vi "WLC Fitting For OneDirectionOnly_Slope_YCC.vi"() -> ()   [LabVIEW 2014]
uses:
  SubVI/WLC-Fitting Cluster.ctl
  <vilib>/gmath/NI_Gmath.lvlib
  <vilib>/gmath/NumericalOptimization/Nonlinear Curve Fit LM formula string.vi
  <vilib>/Utility/file.llb/Write To Spreadsheet File (DBL).vi
  <vilib>/Utility/file.llb/Read From Spreadsheet File (DBL).vi
panel:
  in  "F+U data?":bool
  in  "Ready to Fit":bool
  out "Save to Path":path
  out "best nonlinear fit force":dbl[](array[numeric])
  in  "SaveName":enum16{"ForecExtension Only", "WLC Fitting"}(ring)
  in  "Save Data?":bool
  in  "Finish Fitting":bool
  out "best fit parameters":dbl[](array[numeric])
  in  "initial parameters 2":dbl[](array[numeric])=[40.0, 1150.0]
  in  "Enum":T1(ring)
  in  "initial parameters for fit K":dbl[](array[numeric])=[40.0, 1150.0]
  out "Force":dbl[](array[numeric])
  out "xDNA":dbl[](array[numeric])
  out "Fitting Cluster for indicator":T2={"cr (um)"=0.0, "yr (V)"=0.0, "trap height(nm)"=0.0, "bead radius(nm)"=520.0, "Length offset"=0.0, "Upper Force(pN)"=0.0, "cr shift (nm)"=0.0, "yr shift (mV)"=0.0, "LaserPower (mW)"=0.0, "conversion factor (V/um)"=0.0, "Stiffness (pN/nm)"=0.0154, "xDNA cut outside"=3000.0, "Lower Force(pN)"=5.0}
  in  "OneDirectionOnly?":bool=TRUE
  in  "Fitting Cluster for contorl":T3={"cr (um)"=0.0, "yr (V)"=0.0, "trap height(nm)"=300.0, "bead radius(nm)"=515.0, "Length offset"=0.0, "conversion factor (V/um)"=0.0, "Force constant (pN/nm)"=0.0154, "Force offset"=5.0, "cr shift (nm)"=0.0, "yr shift (mV)"=0.0, "LaserPower (mW)"=30.0, "Cf. Calib. Array"=[0.10341, -0.29934], "Stiffness Calib. array"=[0.0034, -0.00514]}
  in  "Tab Control":T4(tab)
  out "Stage-QPD Graph":T5(graph)
  out "Extension-Force Graph":cluster{"xDNA":dbl[], "Force":dbl[]}(graph)
  out "Extension-Force and WLC Graph":cluster{"xDNA":dbl[], "Force":dbl[]}[](graph)
  out "Cut Stage Position (um)":dbl[](array[numeric])
  out "Cut QPD (V)":dbl[](array[numeric])
  in  "Delete Outside Signal?":bool
  out "QPD signal (V)":dbl[](array[numeric])
  out "Stage Positions (um)":dbl[](array[numeric])
  in  "Load Stage-QPD data":path
  in  "QPD":dbl[](array[numeric])
  in  "Stage":dbl[](array[numeric])
  in  "T=Read data mode?\nF=Real time fit":bool=TRUE
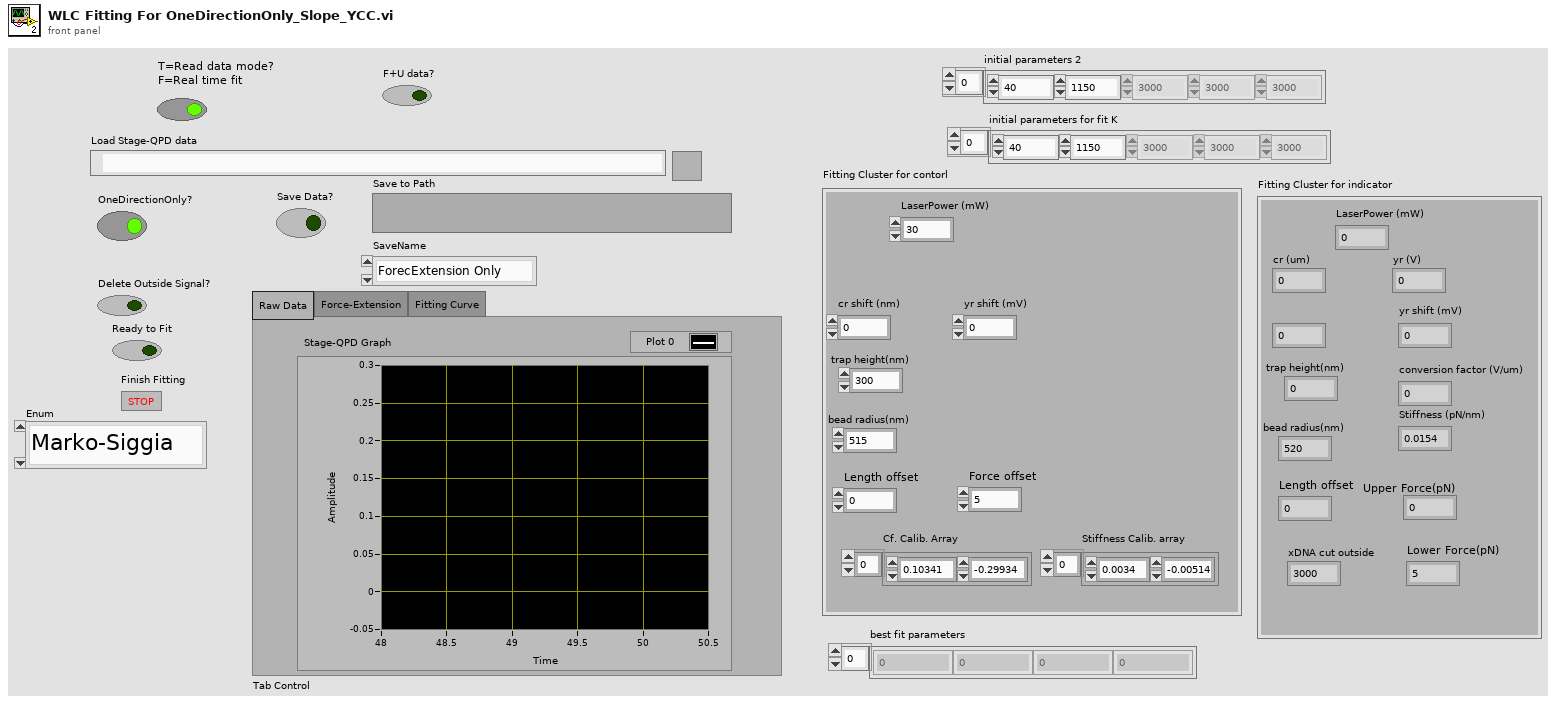
[diagram p1: front panel]
types:
  T1 = enum16{"Marko-Siggia", "modified Marko", "eWLC", "eWLC-modified M-S", "K fit eWLC-modified M-S"}
  T2 = typedef "WLC-Fitting Cluster.ctl" = cluster{"cr (um)":dbl, "yr (V)":dbl, "trap height(nm)":dbl, "bead radius(nm)":dbl, "Length offset":dbl, "Upper Force(pN)":dbl, "cr shift (nm)":dbl, "yr shift (mV)":dbl, "LaserPower (mW)":dbl, "conversion factor (V/um)":dbl, "Stiffness (pN/nm)":dbl, "xDNA cut outside":dbl, "Lower Force(pN)":dbl}
  T3 = typedef "WLC-Fitting Cluster.ctl" = cluster{"cr (um)":dbl, "yr (V)":dbl, "trap height(nm)":dbl, "bead radius(nm)":dbl, "Length offset":dbl, "conversion factor (V/um)":dbl, "Force constant (pN/nm)":dbl, "Force offset":dbl, "cr shift (nm)":dbl, "yr shift (mV)":dbl, "LaserPower (mW)":dbl, "Cf. Calib. Array":dbl[], "Stiffness Calib. array":dbl[]}
  T4 = enum32{"Raw Data", "Force-Extension", "Fitting Curve"}
  T5 = cluster{"Sorted Stage Position (um)":dbl[], "Sorted QPD (V)":dbl[]}[]
  T6 = cluster{"model":string, "Parameters":string[], "x":string}
  T7 = cluster{"Stage Positions (um)":dbl[], "QPD signal (V)":dbl[]}
  T8 = cluster{"Position Array Out":dbl[], "QPD signal Out":dbl[]}
  T9 = cluster{"Stage Positions (um)":dbl[], "QPD signal (V)":dbl[]}[]
  T10 = cluster{"Unfolded-xDNA":dbl[], "Unfolded-Force":dbl[]}
  T11 = cluster{"xDNA":dbl[], "best nonlinear fit":dbl[]}
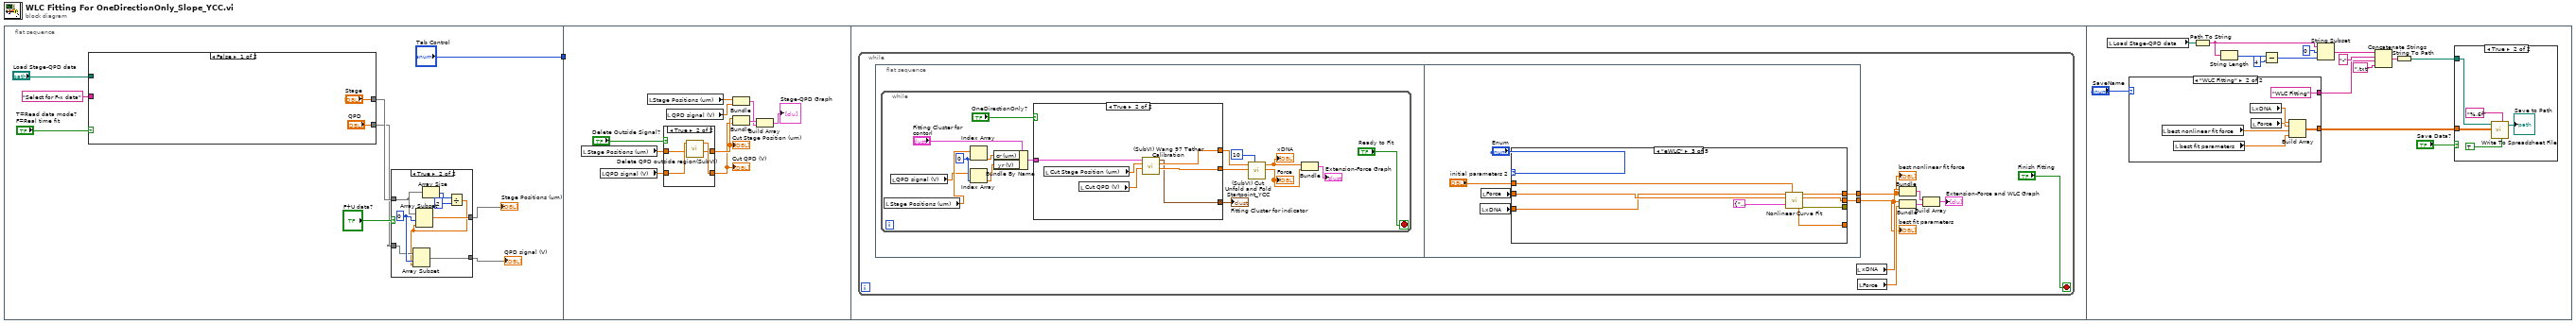
[diagram p0: block diagram]
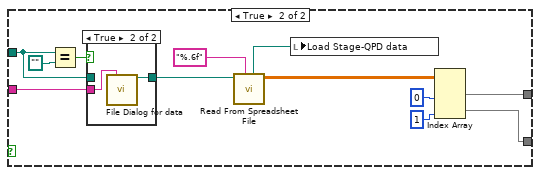
[diagram p3: hidden frame]
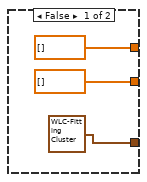
[diagram p6: hidden frame]
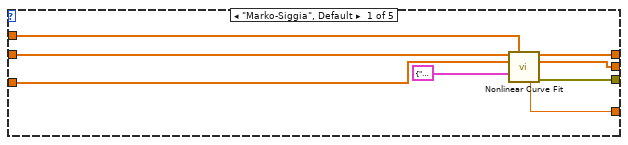
[diagram p7: hidden frame]
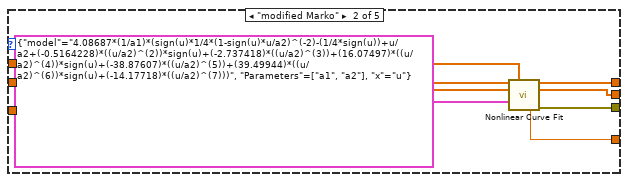
[diagram p8: hidden frame]
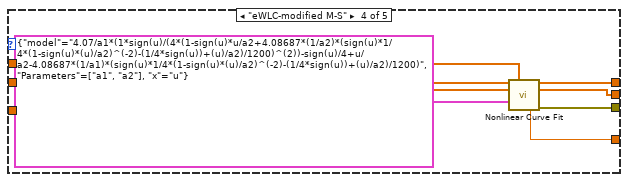
[diagram p9: hidden frame]
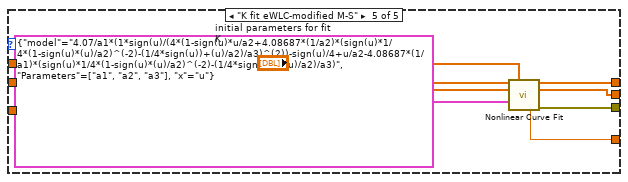
[diagram p10: hidden frame]
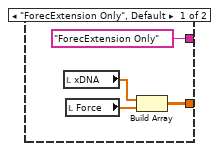
[diagram p11: hidden frame]
diagram:
  n1 = flat-sequence {
    tunnel: ["Tab Control"] -> w1
    tunnel: w1 -> [_]
    frame #0 {
      n2 = case shown="False" "T=Read data mode?\nF=Real time fit" {
        tunnel: ["QPD" w30] -> w4
        tunnel: ["Stage" w31] -> w5
        tunnel: "Select for F-x data" ("default name") -> [_ w27]
        tunnel: "Load Stage-QPD data" -> [_ w24]
        frame False {
        }
        frame True {
          n3 = Equal?(x=w24, y=path "") -> (x = y?=w25:bool)
          n4 = case shown="True" w25 {
            tunnel: [w35 w36] -> w28
            tunnel: w27 -> [_ w37]
            tunnel: w24 -> [w35 _]
            frame False {
            }
            frame True {
              n5 = call "File Dialog for data"("prompt"=w37) -> ("selected path"=w36:path)  [unwired: 11 in, 3 out]
            }
          }
          n6 = call-poly <vilib>:"Read From Spreadsheet File.vi"("format (%.3f)"="%.6f", "file path (dialog if empty)"=w28) -> ("all rows"=w34:dbl[][], "new file path (Not A Path if cancelled)"=w23:path)  [unwired: 5 in, 3 out]
          n7 = local write "Load Stage-QPD data"(w23) -> ()
          n8 = Index Array(array=w34, index (col) #1=0 ("disabled index (col)"), index (col) #2=1 ("index (col)")) -> (element #1=w31:dbl[], element #2=w30:dbl[])  [unwired: 2 in]
        }
      }
      n9 = case shown="True" "F+U data?" {
        tunnel: w5 -> [w12 w20]
        tunnel: w4 -> [w11 w15]
        tunnel: [w12 w17] -> w3
        tunnel: [w11 w13] -> w2
        frame False {
        }
        frame True {
          w16 = 0 ("index")
          n10 = Array Size(array=w20) -> (size(s)=w19:i32)
          n11 = Divide(x=w19, y=2) -> (x/y=w14:dbl)
          n12 = Array Subset(array=w15, index=w16, length=w14) -> (w13:dbl[])
          n13 = Array Subset(array=w20, index=w16, length=w14) -> (w17:dbl[])
        }
      }
      "Stage Positions (um)" <- w3
      "QPD signal (V)" <- w2
    }
    frame #1 {
      n14 = local read "Stage Positions (um)"() -> (w46:dbl[])
      n15 = local read "QPD signal (V)"() -> (w45:dbl[])
      n16 = local read "Stage Positions (um)"() -> (w44:dbl[])
      n17 = case shown="True" "Delete Outside Signal?" {
        tunnel: w45 -> [w49 w53]
        tunnel: w46 -> [w48 w52]
        tunnel: [w49 w51] -> w38
        tunnel: [w48 w50] -> w39
        frame False {
        }
        frame True {
          n18 = call "Delete QPD outside region(SubVI).vi"("Position Array In"=w52, "QPD signal In"=w53) -> ("Position Array Out"=w50:dbl[], "QPD signal Out"=w51:dbl[])  [unwired: 8 in]
        }
      }
      "Cut QPD (V)" <- w38
      "Cut Stage Position (um)" <- w39
      n19 = local read "QPD signal (V)"() -> (w43:dbl[])
      n20 = Bundle("Stage Positions (um)"=w44, "QPD signal (V)"=w43) -> (w41:T7)  [unwired: 1 in]
      n21 = Bundle("Position Array Out"=w39, "QPD signal Out"=w38) -> (w42:T8)  [unwired: 1 in]
      n22 = Build Array(w42, w41) -> (→"Stage-QPD Graph":T9)
    }
    frame #2 {
      n23 = while {
        stop <- "Finish Fitting" stop-if-true
        n24 = flat-sequence {
          tunnel: [w88] -> w55
          tunnel: [w87] -> w54
          frame #0 {
            n25 = while {
              stop <- "Ready to Fit" stop-if-true
              w75 = 0 ("index")
              n26 = local read "Stage Positions (um)"() -> (w64:dbl[])
              n27 = local read "QPD signal (V)"() -> (w63:dbl[])
              n28 = Index Array(array=w64, index=w75) -> (element=w72:dbl)
              n29 = Index Array(array=w63, index=w75) -> (element=w62:dbl)
              n30 = Bundle By Name(cluster="Fitting Cluster for contorl", "cr (um)"=w72, "yr (V)"=w62) -> (w74:T3)
              n31 = case shown="True" "OneDirectionOnly?" {
                tunnel: w74 -> [_ w86]
                tunnel: [T2 {"cr (um)"=0.0, "yr (V)"=0.0, "trap height(nm)"=0.0, "bead radius(nm)"=520.0, "Length offset"=0.0, "Upper Force(pN)"=0.0, "cr shift (nm)"=0.0, "yr shift (mV)"=0.0, "LaserPower (mW)"=0.0, "conversion factor (V/um)"=0.0, "Stiffness (pN/nm)"=0.0154, "xDNA cut outside"=3000.0, "Lower Force(pN)"=5.0} ("Fitting Cluster for contorl") w81] -> w73
                tunnel: [dbl[] [] ("xDNA") w83] -> w68
                tunnel: [dbl[] [] ("Force") w82] -> w67
                frame False {
                }
                frame True {
                  n32 = local read "Cut Stage Position (um)"() -> (w85:dbl[])
                  n33 = local read "Cut QPD (V)"() -> (w84:dbl[])
                  n34 = call "(SubVI) Wang 97 Tether Calibration.vi"("QPD signal"=w84, "Stage Position"=w85, "Fitting Cluster"=w86) -> ("Force"=w82:dbl[], "xDNA"=w83:dbl[], "output cluster"=w81:T2)  [unwired: 2 in]
                }
              }
              "Fitting Cluster for indicator" <- w73
              n35 = call "(SubVI) Cut Unfold and Fold Startpoint_YCC.vi"("number to cut"=10, "Unfolded-Force"=w67, "Unfolded-xDNA"=w68) -> ("Unfolded-Force"=w65:dbl[], "Unfolded-xDNA"=w66:dbl[])  [unwired: 5 in, 2 out]
              "xDNA" <- w66
              "Force" <- w65
              n36 = Bundle("Unfolded-xDNA"=w66, "Unfolded-Force"=w65) -> (→"Extension-Force Graph":T10)  [unwired: 1 in]
            }
          }
          frame #1 {
            n37 = local read "xDNA"() -> (w90:dbl[])
            n38 = local read "Force"() -> (w91:dbl[])
            n39 = case shown="\"eWLC\"" "Enum" {
              tunnel: "initial parameters 2" -> [w94 w107 w113 w123 _]
              tunnel: w91 -> [w99 w105 w115 w121 w131]
              tunnel: w90 -> [w93 w106 w114 w122 w130]
              tunnel: [w98 w102 w111 w117 w125] -> w88
              tunnel: [w97 w103 w112 w118 w126] -> w87
              tunnel: [w96 w104 w110 w119 w127] -> _
              tunnel: [w95 w101 w109 w120 w128] -> _
              frame "Marko-Siggia", Default {
                n40 = call-poly <vilib>:"Nonlinear Curve Fit.vi"("Y"=w99, "initial parameters"=w94, "X"=w93, "model description"=T6 {"model"="4.08687*(1/a1)*(sign(u)*1/4*(1-sign(u)*u/a2)^(-2)-(1/4*sign(u))+u/a2)", "Parameters"=["a1", "a2"], "x"="u"}) -> ("best nonlinear fit"=w98:dbl[], "best fit parameters"=w97:dbl[], "residue"=w95:dbl, "error out"=w96:errorcluster)  [unwired: 3 in, 5 out]
              }
              frame "modified Marko" {
                n41 = call-poly <vilib>:"Nonlinear Curve Fit.vi"("Y"=w105, "initial parameters"=w107, "X"=w106, "model description"=T6 {"model"="4.08687*(1/a1)*(sign(u)*1/4*(1-sign(u)*u/a2)^(-2)-(1/4*sign(u))+u/a2+(-0.5164228)*((u/a2)^(2))*sign(u)+(-2.737418)*((u/a2)^(3))+(16.07497)*((u/a2)^(4))*sign(u)+(-38.87607)*((u/a2)^(5))+(39.49944)*((u/a2)^(6))*sign(u)+(-14.17718)*((u/a2)^(7)))", "Parameters"=["a1", "a2"], "x"="u"}) -> ("best nonlinear fit"=w102:dbl[], "best fit parameters"=w103:dbl[], "residue"=w101:dbl, "error out"=w104:errorcluster)  [unwired: 3 in, 5 out]
              }
              frame "eWLC" {
                n42 = call-poly <vilib>:"Nonlinear Curve Fit.vi"("Y"=w114, "initial parameters"=w113, "X"=w115, "model description"=T6 {"model"="a2*(1*sign(u)-sign(u)*1/2*(4.07/u/a1)^(0.5)+sign(u)*u/1200)", "Parameters"=["a1", "a2"], "x"="u"}) -> ("best nonlinear fit"=w111:dbl[], "best fit parameters"=w112:dbl[], "residue"=w109:dbl, "error out"=w110:errorcluster)  [unwired: 3 in, 5 out]
              }
              frame "eWLC-modified M-S" {
                n43 = call-poly <vilib>:"Nonlinear Curve Fit.vi"("Y"=w121, "initial parameters"=w123, "X"=w122, "model description"=T6 {"model"="4.07/a1*(1*sign(u)/(4*(1-sign(u)*u/a2+4.08687*(1/a2)*(sign(u)*1/4*(1-sign(u)*(u)/a2)^(-2)-(1/4*sign(u))+(u)/a2)/1200)^(2))-sign(u)/4+u/a2-4.08687*(1/a1)*(sign(u)*1/4*(1-sign(u)*(u)/a2)^(-2)-(1/4*sign(u))+(u)/a2)/1200)", "Parameters"=["a1", "a2"], "x"="u"}) -> ("best nonlinear fit"=w117:dbl[], "best fit parameters"=w118:dbl[], "residue"=w120:dbl, "error out"=w119:errorcluster)  [unwired: 7 in, 1 out]
              }
              frame "K fit eWLC-modified M-S" {
                n44 = call-poly <vilib>:"Nonlinear Curve Fit.vi"("Y"=w131, "initial parameters"="initial parameters for fit K", "X"=w130, "model description"=T6 {"model"="4.07/a1*(1*sign(u)/(4*(1-sign(u)*u/a2+4.08687*(1/a2)*(sign(u)*1/4*(1-sign(u)*(u)/a2)^(-2)-(1/4*sign(u))+(u)/a2)/a3)^(2))-sign(u)/4+u/a2-4.08687*(1/a1)*(sign(u)*1/4*(1-sign(u)*(u)/a2)^(-2)-(1/4*sign(u))+(u)/a2)/a3)", "Parameters"=["a1", "a2", "a3"], "x"="u"}) -> ("best nonlinear fit"=w125:dbl[], "best fit parameters"=w126:dbl[], "residue"=w128:dbl, "error out"=w127:errorcluster)  [unwired: 7 in, 1 out]
              }
            }
          }
        }
        n45 = local read "xDNA"() -> (w60:dbl[])
        n46 = local read "Force"() -> (w59:dbl[])
        n47 = Bundle("xDNA"=w60, "best nonlinear fit"=w55) -> (w58:T11)  [unwired: 1 in]
        n48 = Bundle("xDNA"=w60, "Force"=w59) -> (w57:cluster{"xDNA":dbl[], "Force":dbl[]})  [unwired: 1 in]
        n49 = Build Array(w58, w57) -> (→"Extension-Force and WLC Graph":cluster{"xDNA":dbl[], "Force":dbl[]}[])
        "best nonlinear fit force" <- w55
        "best fit parameters" <- w54
      }
    }
    frame #3 {
      n50 = local read "Load Stage-QPD data"() -> (w147:path)
      n51 = case shown="\"WLC Fitting\"" "SaveName" {
        tunnel: ["ForecExtension Only" ("string") "WLC Fitting" ("string")] -> w137
        tunnel: [w148 w152] -> w133
        frame "ForecExtension Only", Default {
          n52 = local read "xDNA"() -> (w150:dbl[])
          n53 = local read "Force"() -> (w149:dbl[])
          n54 = Build Array(w150, w149) -> (w148:dbl[][])
        }
        frame "WLC Fitting" {
          n55 = local read "best nonlinear fit force"() -> (w154:dbl[])
          n56 = local read "best fit parameters"() -> (w153:dbl[])
          n57 = local read "xDNA"() -> (w156:dbl[])
          n58 = local read "Force"() -> (w155:dbl[])
          n59 = Build Array(w156, w155, w154, w153) -> (w152:dbl[][])
        }
      }
      n60 = Path To String(path=w147) -> (string=w145:string)
      n61 = String Length(string=w145) -> (length=w144:i32)
      n62 = Subtract(x=w144, y=4) -> (x-y=w141:i32)
      n63 = String Subset(string=w145, offset (0)=0, length (rest)=w141) -> (substring=w140:string)
      n64 = Concatenate Strings(w140, "-" ("string"), w137, ".txt" ("string")) -> (w135:string)
      n65 = String To Path(string=w135) -> (path=w134:path)
      n66 = case shown="True" "Save Data?" {
        tunnel: w134 -> [_ w162]
        tunnel: w133 -> [_ w161]
        frame False {
        }
        frame True {
          n67 = call-poly <vilib>:"Write To Spreadsheet File.vi"("transpose? (no:F)"=TRUE, "format (%.3f)"="%.6f", "2D data"=w161, "file path (dialog if empty)"=w162) -> ("new file path (Not A Path if cancelled)"=→"Save to Path":path)  [unwired: 4 in]
        }
      }
    }
  }
